vi "SCADA.vi"() -> ()   [LabVIEW 2013]
uses:
  <vilib>/Instr/_visa.llb/VISA Configure Serial Port (Instr).vi
  <vilib>/addons/control/pid/pid.llb/PID (DBL).vi
  <vilib>/addons/control/pid/NI_PID_pid.lvlib
panel:
  out "Numeric":i32
  in  "Reinitialize PID":bool
  in  "Square   Senoide":bool
  in  "Manual":dbl
  in  "Setpoint\n\nManual       Auto":bool
  out "SP (%)":u8(slide) scale=0.0..100.0
  out "CV (%)":u8(slide) scale=0.0..100.0
  out "PV (%)":u8(slide) scale=0.0..100.0
  in  "PWM Write":bool
  out "CV (PWM)":dynamicdata(graph)
  out "SP x  PV (Hz)":dynamicdata(graph)
  in  "dt (s)":dbl=-1.0 format="%.3f"
  in  "PID gains":T1={"proportional gain (Kc)"=1.0, "integral time (Ti, min)"=0.01, "derivative time (Td, min)"=0.0} {"derivative time (Td, min)" format="%.3f"; "integral time (Ti, min)" format="%.3f"; "proportional gain (Kc)" format="%.3f"}
  in  "Serial Port":refnum<visa-resource-name>
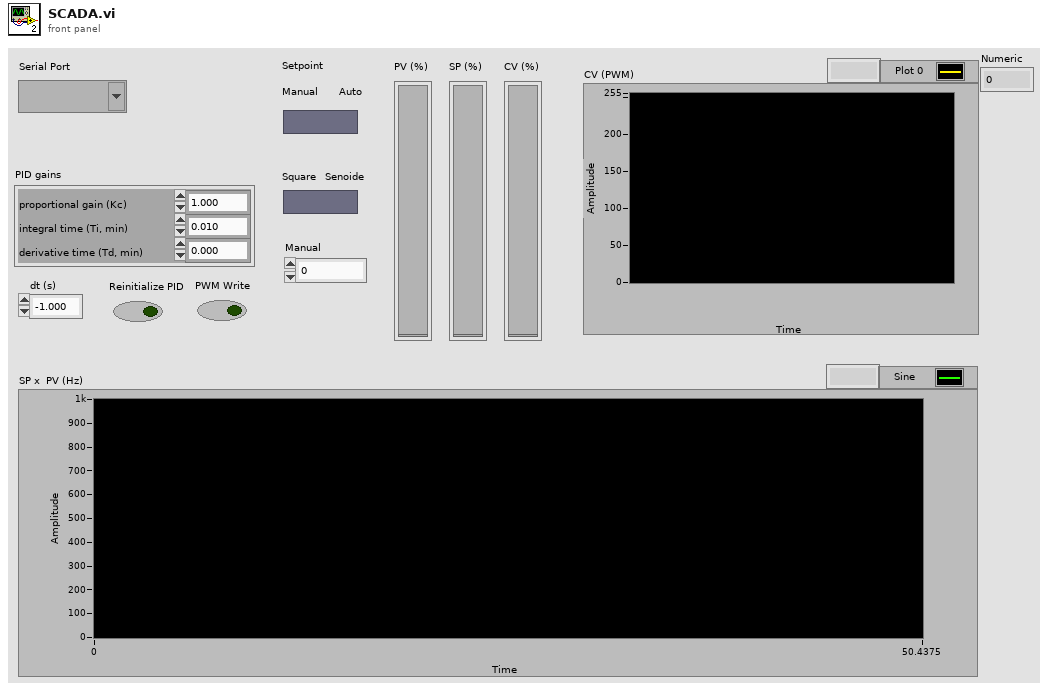
[diagram p1: front panel]
types:
  T1 = cluster{"proportional gain (Kc)":dbl, "integral time (Ti, min)":dbl, "derivative time (Td, min)":dbl}
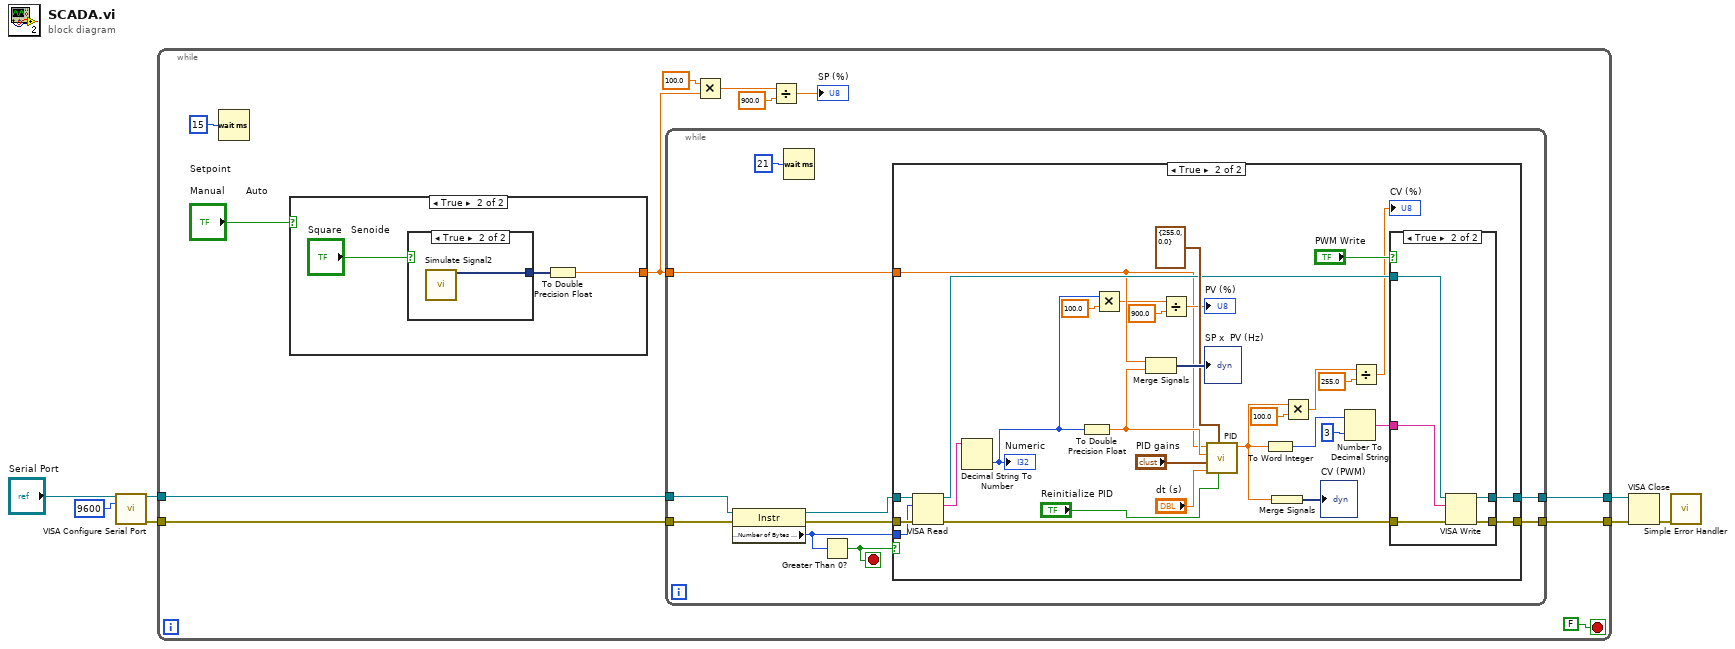
[diagram p0: block diagram]
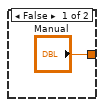
[diagram p2: hidden frame]
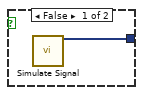
[diagram p3: hidden frame]
diagram:
  n1 = call-poly "VISA Configure Serial Port"("VISA resource name"="Serial Port", "baud rate (9600)"=u32 9600) -> ("VISA resource name out"=w2:refnum<visa-resource-name>, "error out"=w1:errorcluster)  [unwired: 12 in]
  n2 = while {
    tunnel: [w17] -> w4
    tunnel: [w16] -> w3
    tunnel: w2 -> [w15]
    tunnel: w1 -> [w14]
    stop <- FALSE stop-if-true
    n3 = Wait (ms)(milliseconds to wait=u32 15) -> ()  [unwired: 1 out]
    n4 = case shown="True" "Setpoint\n\nManual       Auto" {
      tunnel: ["Manual" w21] -> w8
      frame False {
      }
      frame True {
        n5 = case shown="True" "Square   Senoide" {
          tunnel: [w24 w25] -> w22
          frame False {
            n6 = call "Simulate Signal"() -> ("Square"=w24:dynamicdata)  [unwired: 14 in, 1 out]
          }
          frame True {
            n7 = call "Simulate Signal2"() -> ("Sine"=w25:dynamicdata)  [unwired: 14 in, 1 out]
          }
        }
        n8 = To Double Precision Float(number=w22) -> (double precision float=w21:dbl)
      }
    }
    n9 = while {
      tunnel: [w30] -> w17
      tunnel: [w29] -> w16
      tunnel: w15 -> [w28]
      tunnel: w14 -> [w27]
      tunnel: w8 -> [w26]
      stop <- w31 stop-if-true
      n10 = property class="Instr"(reference=w28, error in=w27) -> (reference out=w32:refnum<visa-resource-name>, error out=w33:errorcluster, "Serial Settings:Number of Bytes at Serial Port"=w34:u32)
      n11 = Wait (ms)(milliseconds to wait=u32 21) -> ()  [unwired: 1 out]
      n12 = Greater Than 0?(x=w34) -> (x > 0?=w31:bool)
      n13 = case shown="True" w31 {
        tunnel: w32 -> [w37 w67]
        tunnel: w33 -> [w36 w66]
        tunnel: w34 -> [_ w65]
        tunnel: [w37 w53] -> w30
        tunnel: [w36 w51] -> w29
        tunnel: w26 -> [_ w41]
        frame False {
        }
        frame True {
          n14 = VISA Read(VISA resource name=w67, byte count=w65, error in (no error)=w66) -> (VISA resource name out=w56:refnum<visa-resource-name>, read buffer=w62:string, error out=w55:errorcluster)  [unwired: 1 out]
          n15 = Decimal String To Number(string=w62) -> (number=w38:i32)  [unwired: 2 in, 1 out]
          "Numeric" <- w38
          n16 = To Double Precision Float(number=w38) -> (double precision float=w42:dbl)
          n17 = Multiply(x=w38, y=100.0) -> (x*y=w39:dbl)
          n18 = Merge Signals(w41, w42) -> (→"SP x  PV (Hz)":dynamicdata)
          n19 = Divide(x=w39, y=900.0) -> (x/y=→"PV (%)":dbl)
          n20 = call-poly <vilib>:"PID.vi"("reinitialize? (F)"="Reinitialize PID", "output range"=cluster{"output high":dbl, "output low":dbl} {"output high"=255.0, "output low"=0.0}, "dt (s)"="dt (s)", "PID gains"="PID gains", "process variable"=w42, "setpoint"=w41) -> ("output"=w44:dbl)  [unwired: 4 in, 1 out]
          n21 = To Word Integer(number=w44) -> (16bit integer=w57:i16)
          n22 = Merge Signals(w44) -> (→"CV (PWM)":dynamicdata)
          n23 = Multiply(x=w44, y=100.0) -> (x*y=w49:dbl)
          n24 = Number To Decimal String(number=w57, width (-)=i16 3) -> (decimal integer string=w54:string)
          n25 = Divide(x=w49, y=255.0) -> (x/y=→"CV (%)":dbl)
          n26 = case shown="True" "PWM Write" {
            tunnel: w56 -> [w69 w74]
            tunnel: w55 -> [w68 w73]
            tunnel: w54 -> [_ w72]
            tunnel: [w69 w71] -> w53
            tunnel: [w68 w70] -> w51
            frame False {
            }
            frame True {
              n27 = VISA Write(VISA resource name=w74, write buffer=w72, error in (no error)=w73) -> (VISA resource name out=w71:refnum<visa-resource-name>, error out=w70:errorcluster)  [unwired: 1 out]
            }
          }
        }
      }
    }
    n28 = Multiply(x=100.0, y=w8) -> (x*y=w12:dbl)
    n29 = Divide(x=w12, y=900.0) -> (x/y=→"SP (%)":dbl)
  }
  n30 = VISA Close(VISA resource name=w4, error in (no error)=w3) -> (error out=w6:errorcluster)
  n31 = call <vilib>:"Simple Error Handler.vi"("error in (no error)"=w6) -> ()  [unwired: 4 in, 5 out]
